vi "E4_readDataAndCutBuffer.vi"(8 "error in (no error)":errorcluster, 9 "channelsToRead":i16, 10 "Numeric":i16, 11 "RefNum in":refnum<vi>) -> (0 "error out":errorcluster, 2 "Array":i16[](array[numeric]), 3 "function return":u32)   [LabVIEW 2021]
uses:
  <userlib>/er4commlib_labview/er4commlib_labview.lvlib
panel:
  out "reversed array":i16[](array[numeric])
  out "size(s)":i32
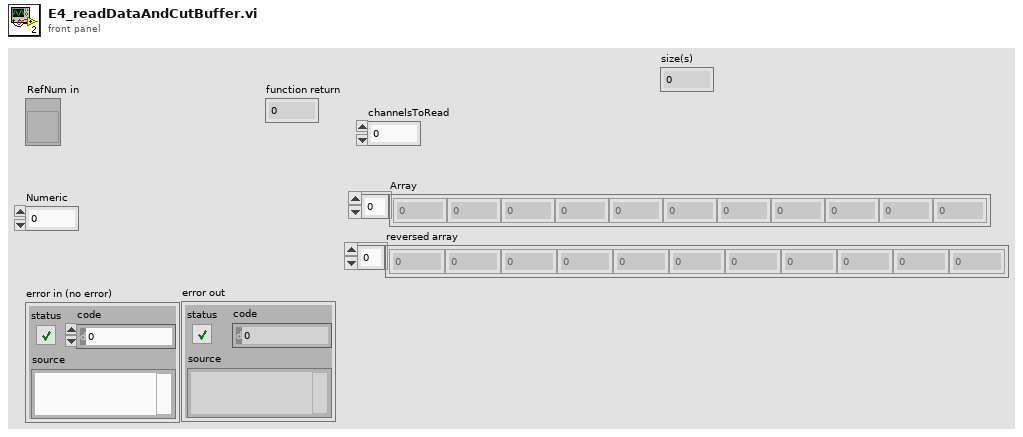
[diagram p1: front panel]
types:
  T1 = enum16{"big-endian, network order", "native, host order", "little-endian"}
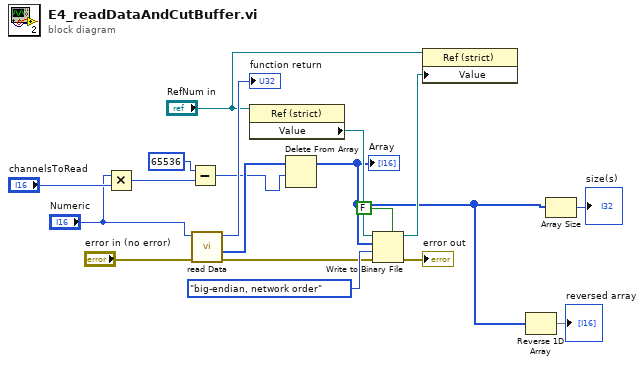
[diagram p0: block diagram]
diagram:
  n1 = Multiply(x="Numeric", y="channelsToRead") -> (x*y=w8:i16)
  n2 = Subtract(x=65536, y=w8) -> (x-y=w2:i32)
  n3 = call <userlib>:"read Data.vi"("error in (no error)"="error in (no error)", "dataToRead"="Numeric") -> ("error out"=w15:errorcluster, "buffer out"=w10:i16[], "function return"=→"function return":u32)  [unwired: 6 in, 1 out]
  n4 = property class="Ref (strict)"(reference="RefNum in") -> ("Value"=w14:refnum<file>)  [unwired: 1 in, 2 out]
  n5 = Delete From Array(array=w10, length=w2) -> (array with subset deleted=w4:i16[])  [unwired: 1 in, 1 out]
  "Array" <- w4
  n6 = Write to Binary File(file (use dialog)=w14, data=w4, error in=w15, 5:FALSE ("prepend array or string size? (T)"), 9:T1."big-endian, network order" ("byte order (0:big-endian, network order)")) -> (refnum out=w17:refnum<file>, error out=→"error out":errorcluster)  [unwired: 1 in, 1 out]
  n7 = property class="Ref (strict)"(reference="RefNum in", "Value"=w17) -> ()  [unwired: 1 in, 2 out]
  n8 = Reverse 1D Array(array=w4) -> (reversed array=→"reversed array":i16[])
  n9 = Array Size(array=w4) -> (size(s)=→"size(s)":i32)
